vi "setEnableDhcpClient.vi"(8 "error":errorcluster, 10 "enable":bool=TRUE, 11 "connection ID":refnum<k5>) -> (0 "error out":errorcluster, 3 "connection ID out":refnum<k5>)   [LabVIEW 2016, in "amc_api.lvlib"]
doc: "Enables or disables DHCP client."
uses:
  amc_api.lvlib
panel:
  out "jsonRespIn":string
  out "JSON-response":string="{\"jsonrpc\":\"2.0\",\"method\":\"\",\"params\":[5,1.245,true,\"name\"],\"id\":\"1\"}"
  out "JSON request":string
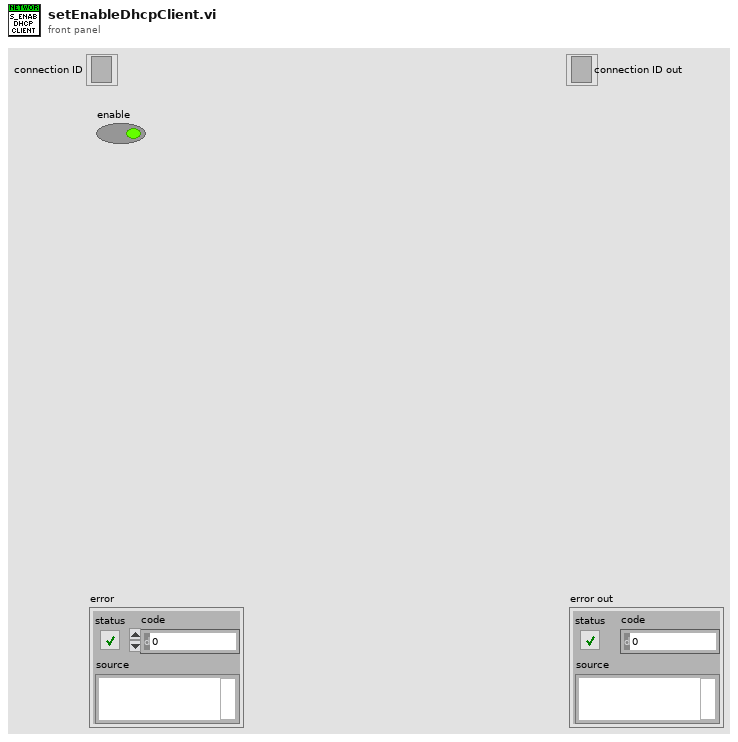
[diagram p1: front panel]
types:
  T1 = cluster{"jsonrpc":string, "method":string, "params":string[], "id":string, "api":i32, "pid":string}
  T2 = enum16{"Standard", "Buffered", "CRLF", "Immediate"}
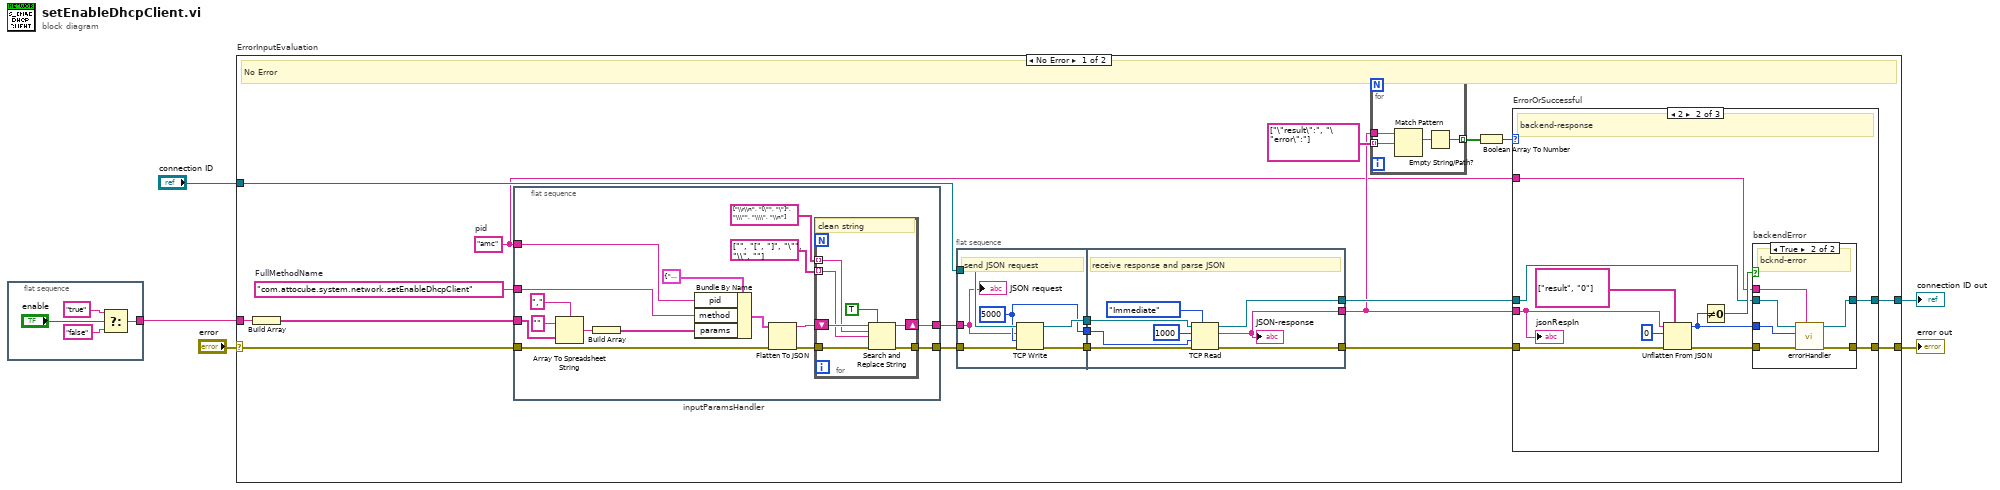
[diagram p0: block diagram]
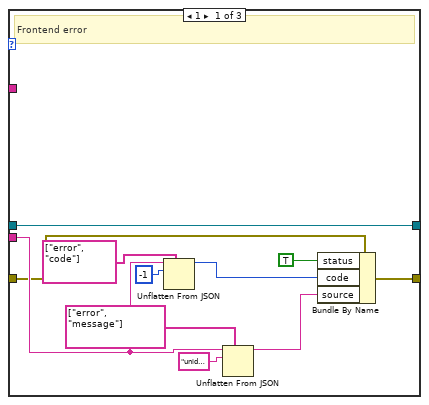
[diagram p2: hidden frame]
diagram:
  n1 = flat-sequence "in_bool" {
    tunnel: [w6] -> w1
    frame #0 {
      n2 = Select(t="true" ("Base"), s="enable", f="false" ("Base")) -> (s? t:f=w6:string)
    }
  }
  n3 = case "ErrorInputEvaluation" shown="No Error" "error" {
    selector: "error" -> [w15 w102]
    tunnel: "connection ID" -> [w25 w103]
    tunnel: [w17 w102] -> w4
    tunnel: [w18 w103] -> w3
    tunnel: w1 -> [w10 _]
    frame No Error {
      w11 = "amc"  # pid
      w16 = "com.attocube.system.network.setEnableDhcpClient"  # FullMethodName
      # "No Error"
      n4 = Build Array ("ParametersArrayString")(w10) -> (w14:string[])
      n5 = flat-sequence "inputParamsHandler" {
        tunnel: [w34] -> w13
        tunnel: w14 -> [w40]
        tunnel: w15 -> [w39]
        tunnel: [w36] -> w12
        tunnel: w16 -> [w30]
        tunnel: w11 -> [w29]
        frame #0 {
          n6 = Array To Spreadsheet String(delimiter (Tab)=",", array=w40, 3:"" ("format string")) -> (spreadsheet string=w42:string)
          n7 = Build Array "Build Array"(w42) -> (w31:string[])
          n8 = Bundle By Name(cluster=T1 {"jsonrpc"="2.0", "method"="com.attocube.amc.res.setRESReadOutFreq", "params"=[], "id"="1", "api"=2, "pid"=""}, "pid"=w29, "method"=w30, "params"=w31) -> (w41:T1)
          n9 = Flatten To JSON(anything=w41, error in (no error)=w39) -> (JSON string=w35:string, 11:w37:errorcluster)  [unwired: 1 in]
          n10 = for {
            tunnel: string[] ["\\r\\n", "[\"", "\"]", "\\\"", "\\\\", "\\n"] ("search string") -> [w48] mode=indexing
            tunnel: string[] ["", "[", "]", "\"", "\\", ""] ("replace string (\"\")") -> [w47] mode=indexing
            shift-right: [w50] -> w34
            shift-left: w35 -> [w49]
            tunnel: w37 -> [w46]
            tunnel: [w45] -> w36
            # "clean string"
            n11 = Search and Replace String(replace all?=TRUE ("replace all? (F)"), input string=w49, search string=w48, replace string=w47, error in=w46) -> (result string=w50:string, error out=w45:errorcluster)  [unwired: 3 in, 2 out]
          }
        }
      }
      n12 = flat-sequence {
        tunnel: w25 -> [w93]
        tunnel: [w91] -> w28
        tunnel: [w92] -> w27
        tunnel: w12 -> [w88]
        tunnel: [w90] -> w26
        tunnel: w13 -> [w89]
        tunnel: [w97] -> w21
        tunnel: w28 -> [w99]
        tunnel: w27 -> [w98]
        tunnel: [w95] -> w20
        tunnel: w26 -> [w96]
        tunnel: [w94] -> w19
        frame #0 {
          w90 = 5000 ("timeout ms (25000)")
          # "send JSON request"
          n13 = TCP Write(connection ID=w93, data in=w89, error in (no error)=w88, 9:w90) -> (connection ID out=w91:refnum<k5>, error out=w92:errorcluster)  [unwired: 1 out]
          "JSON request" <- w89
        }
        frame #1 {
          # "receive response and parse JSON"
          n14 = TCP Read(connection ID=w99, bytes to read=1000, error in (no error)=w98, 7:T2."Immediate" ("mode (standard)"), 9:w96) -> (connection ID out=w97:refnum<k5>, data out=w94:string, error out=w95:errorcluster)
          "JSON-response" <- w94
        }
      }
      n15 = for {
        tunnel: string[] ["\"result\":", "\"error\":"] ("path") -> [w54] mode=indexing
        tunnel: [w52] -> w23 mode=indexing
        tunnel: w19 -> [w55]
        n16 = Match Pattern(string=w55, regular expression=w54) -> (match substring=w53:string)  [unwired: 1 in, 3 out]
        n17 = Empty String/Path?(string/path=w53) -> (empty?=w52:bool)
      }
      n18 = Boolean Array To Number(Boolean array=w23) -> (number=w22:u32)
      n19 = case "ErrorOrSuccessful" shown="2" w22 {
        tunnel: w19 -> [w58 w68 _]
        tunnel: w21 -> [w56 w71 w87]
        tunnel: [w56 w70 w87] -> w18
        tunnel: [w59 w69 w86] -> w17
        tunnel: w20 -> [w57 w72 w86]
        tunnel: w11 -> [_ w67 _]
        frame 1 {
          # "Frontend error"
          n20 = Unflatten From JSON(path=string[] ["error", "code"], JSON string=w58, type and defaults=-1) -> (value=w65:i32)  [unwired: 4 in, 1 out]
          n21 = Unflatten From JSON(path=string[] ["error", "message"], JSON string=w58, type and defaults="unidentified error") -> (value=w66:string)  [unwired: 4 in, 1 out]
          n22 = Bundle By Name(cluster=w57, "status"=TRUE, "code"=w65, "source"=w66) -> (w59:errorcluster)
        }
        frame 2 {
          # "backend-response"
          n23 = Unflatten From JSON(path=string[] ["result", "0"], JSON string=w68, type and defaults=0, error in (no error)=w72) -> (value=w77:i32, error out=w75:errorcluster)  [unwired: 3 in]
          n24 = Not Equal To 0?(x=w77) -> (x != 0?=w76:bool)
          n25 = case "backendError" shown="True" w76 {
            tunnel: w77 -> [_ w85]
            tunnel: w75 -> [w79 w84]
            tunnel: [w78 w83] -> w70
            tunnel: [w79 w82] -> w69
            tunnel: w71 -> [w78 w81]
            tunnel: w67 -> [_ w80]
            frame False {
              # "successful"
            }
            frame True {
              # "bcknd-error"
              n26 = call "errorHandler.vi"("pid"=w80, "error in"=w84, "errNbr"=w85, "connection ID"=w81) -> ("error out 2"=w82:errorcluster, "connection ID out"=w83:refnum<k5>)  [unwired: 6 in]
            }
          }
          "jsonRespIn" <- w68
        }
        frame Default {
          # "NoResponse"
        }
      }
    }
    frame Error {
      # "Error"
    }
  }
  "error out" <- w4
  "connection ID out" <- w3
